vi "AlliGator Compute Lifetime Variances.vi"(8 "error in (no error)":errorcluster, 10 "Lifetime Variance Data Array (in)":T2[](array[typedef]), 11 "Slices Definition":T3={"Axis Start"=0.0, "Axis Stop"=0.0, "# Steps"=0, "Step Size"=0.0, "Step Definition"=enum."# Steps", "Upper Percentile"=0.0, "Lower Percentile"=0.0, "Min # Data Points/Slice"=0, "Output Abscissa Statistics Plots"=FALSE, "Bin Location"=enum."Left", "# Elements"=1, "Bootstrap CV's SDV"=FALSE, "# Replicas"=1} {"# Replicas" min=1; "# Elements" min=0; "Min # Data Points/Slice" min=1; "Lower Percentile" min=0.0 max=100.0; "Upper Percentile" min=0.0 max=100.0; "Step Size" min=0.0; "# Steps" min=1}) -> (0 "error out":errorcluster, 1 "Parameter Map Names":string[](array[string]), 2 "Lifetime Variance Data Array (out)":T2[](array[typedef]))   [LabVIEW 2021, in "AlliGator Decay Fit Parameter Map.lvlib"]
uses:
  AlliGator Decay Fit Parameter Map.lvlib
  Camera Noise Influence on Lifetime/Lifetime Variance Data.ctl
  Graphs/XY Graph/XY Graph Sliced Mean & SDV Step Definition.ctl
  Lifetime & Other Parameters/AlliGator Intensity Slice Definition.ctl
  Graphs/XY Graph/XY Graph Sliced CV Abscissa Location.ctl
  AlliGator Lifetime Variance Statistical Test.ctl
  Lifetime & Other Parameters/AlliGator Lifetime & Other Parameters.lvlib
  Graphs/XY Graph/XY Graph Add-Ons.lvlib
panel:
  in  "Variance Statistical Test":T1
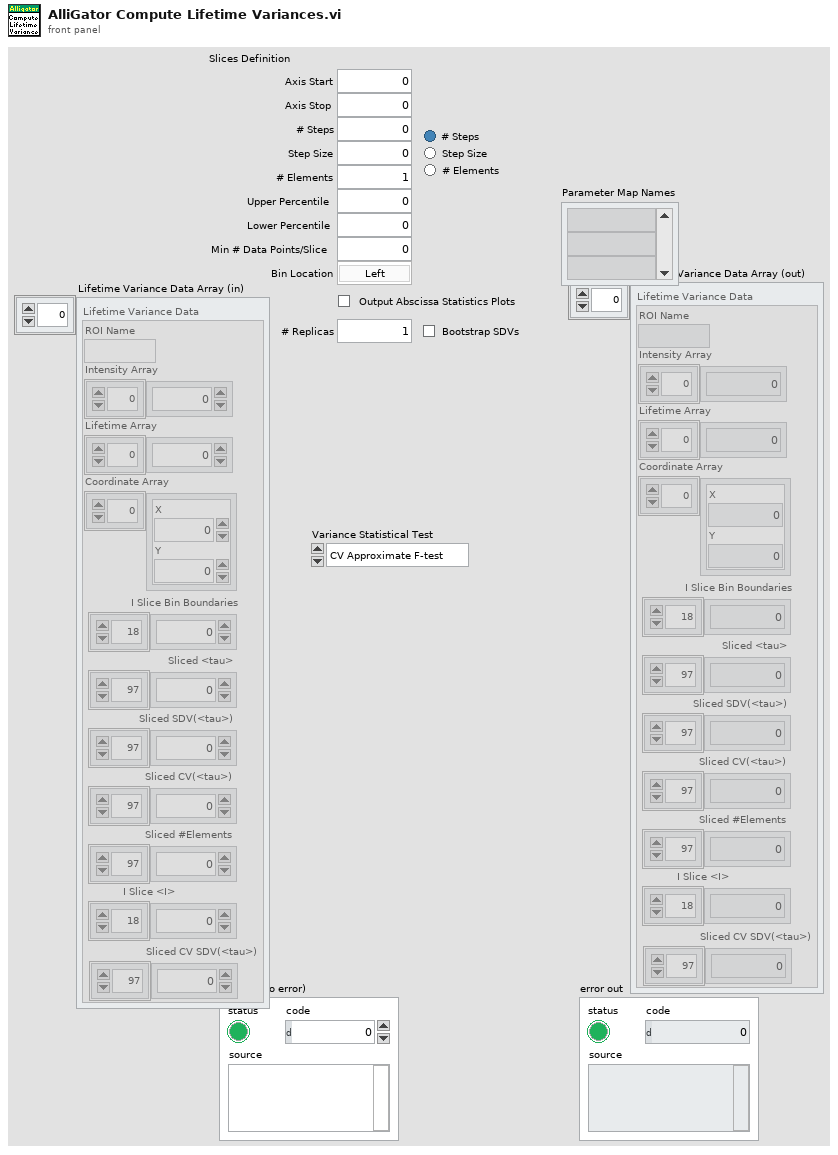
[diagram p1: front panel]
types:
  T1 = typedef "AlliGator Decay Fit Parameter Map.lvlib/AlliGator Lifetime Variance Statistical Test.ctl" = enum16{"CV Approximate F-test", "Variance F-test", "CV Residuals test", "CV Bootstrap SDV Test"}
  T2 = typedef "AlliGator Decay Fit Parameter Map.lvlib/Lifetime Variance Data.ctl" = cluster{"ROI Name":string, "Intensity Array":sgl[], "Lifetime Array":dbl[], "Coordinate Array":cluster{"X":i32, "Y":i32}[], "I Slice Bin Boundaries":dbl[], "Sliced <tau>":dbl[], "Sliced SDV(<tau>)":dbl[], "Sliced CV(<tau>)":dbl[], "Sliced #Elements":i32[], "I Slice <I>":dbl[], "Sliced CV SDV(<tau>)":dbl[]}
  T3 = typedef "XY Graph Add-Ons.lvlib/XY Graph Sliced Mean & SDV Step Definition.ctl" = cluster{"Axis Start":dbl, "Axis Stop":dbl, "# Steps":i32, "Step Size":dbl, "Step Definition":T4, "Upper Percentile":dbl, "Lower Percentile":dbl, "Min # Data Points/Slice":i32, "Output Abscissa Statistics Plots":bool, "Bin Location":T5, "# Elements":i32, "Bootstrap CV's SDV":bool, "# Replicas":i32}
  T4 = typedef "AlliGator Lifetime & Other Parameters.lvlib/AlliGator Intensity Slice Definition.ctl" = enum32{"# Steps", "Step Size", "# Elements"}
  T5 = typedef "XY Graph Add-Ons.lvlib/XY Graph Sliced CV Abscissa Location.ctl" = enum16{"Left", "Center", "Mean", "Right"}
  T6 = cluster{"Intensity Array":sgl[], "Lifetime Array":dbl[]}
  T7 = typedef "AlliGator Decay Fit Parameter Map.lvlib/AlliGator Sliced Analysis Plots.ctl" = cluster{"[<tau>(I)]":T8, "[SDV(tau)(I)]":T8, "[CV(tau)(I)]":T8, "[CV(tau)(I) SDV]":T8, "[N(I)]":T8, "[<I>(I)]":T8, "[SDV(I)(I)]":T8}
  T8 = typedef "XY Graph Add-Ons.lvlib/XY Graph Plot Data.ctl" = cluster{"X Array":dbl[], "Y Array":dbl[]}
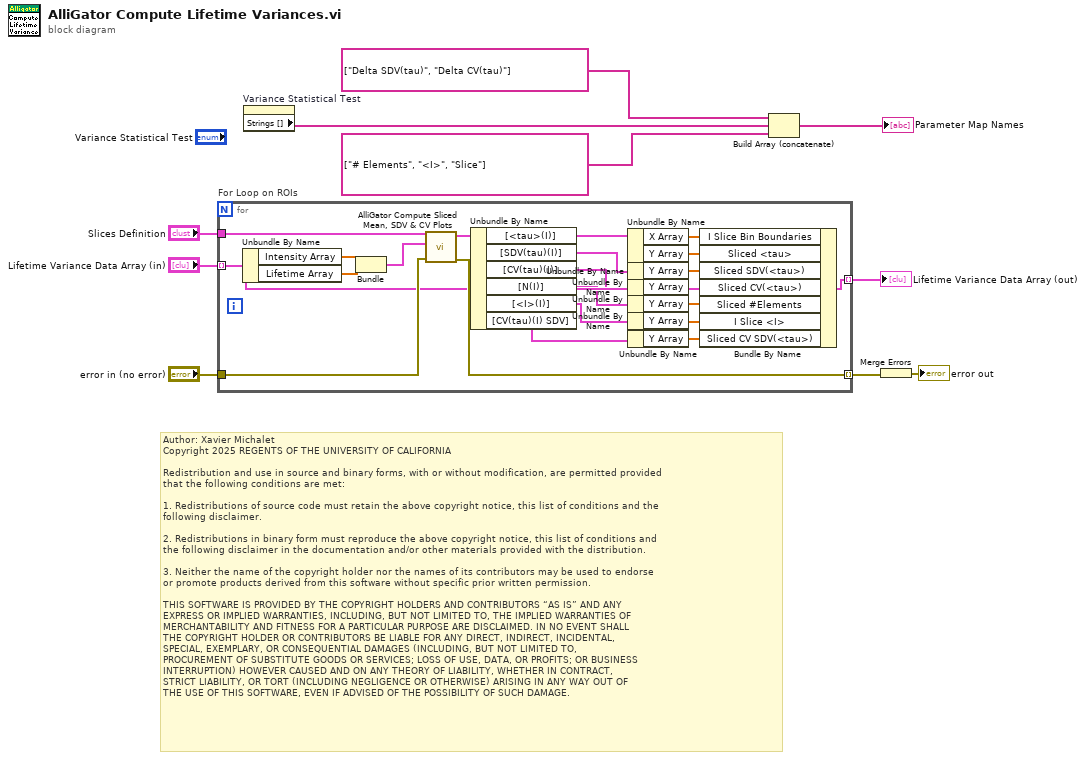
[diagram p0: block diagram]
diagram:
  # "Author: Xavier Michalet\nCopyright 2025 REGENTS OF THE UNIVERSITY OF CALIFORNIA\n\nRedistribution and use in source and binary forms, with or without modification, are permitted provided\nthat the following conditions are met:\n\n1. Redistributions of source code must retain the above copyright notice, this list of conditions and the\nfollowing disclaimer.\n\n2. Redistributions in binary form must reproduce the above copyright notice, this list of conditions and\nthe following disclaimer in the documentation and/or other materials provided with the distribution.\n\n3. Neither the name of the copyright holder nor the names of its contributors may be used to endorse \nor promote products derived from this software without specific prior written permission.\n\nTHIS SOFTWARE IS PROVIDED BY THE COPYRIGHT HOLDERS AND CONTRIBUTORS “AS IS” AND ANY \nEXPRESS OR IMPLIED WARRANTIES, INCLUDING, BUT NOT LIMITED TO, THE IMPLIED WARRANTIES OF\nMERCHANTABILITY AND FITNESS FOR A PARTICULAR PURPOSE ARE DISCLAIMED. IN NO EVENT SHALL\nTHE COPYRIGHT HOLDER OR CONTRIBUTORS BE LIABLE FOR ANY DIRECT, INDIRECT, INCIDENTAL, \nSPECIAL, EXEMPLARY, OR CONSEQUENTIAL DAMAGES (INCLUDING, BUT NOT LIMITED TO, \nPROCUREMENT OF SUBSTITUTE GOODS OR SERVICES; LOSS OF USE, DATA, OR PROFITS; OR BUSINESS\nINTERRUPTION) HOWEVER CAUSED AND ON ANY THEORY OF LIABILITY, WHETHER IN CONTRACT, \nSTRICT LIABILITY, OR TORT (INCLUDING NEGLIGENCE OR OTHERWISE) ARISING IN ANY WAY OUT OF\nTHE USE OF THIS SOFTWARE, EVEN IF ADVISED OF THE POSSIBILITY OF SUCH DAMAGE."
  n1 = for "For Loop on ROIs" {
    tunnel: "Slices Definition" -> [w32]
    tunnel: "Lifetime Variance Data Array (in)" -> [w26] mode=indexing
    tunnel: "error in (no error)" -> [w28]
    tunnel: [w27] -> w7 mode=indexing
    tunnel: [w23] -> w5 mode=indexing
    n2 = Unbundle By Name(w26) -> ("Intensity Array"=w31:sgl[], "Lifetime Array"=w30:dbl[])
    n3 = Bundle("Intensity Array"=w31, "Lifetime Array"=w30) -> (w29:T6)  [unwired: 1 in]
    n4 = call "AlliGator Compute Sliced Mean, SDV & CV Plots.vi"("error in (no error)"=w28, "tau(I) Plot"=w29, "Slices Definition"=w32) -> ("error out"=w27:errorcluster, "Result Plots Cluster"=w22:T7)  [unwired: 5 in, 2 out]
    n5 = Unbundle By Name(w22) -> ("[<tau>(I)]"=w21:T8, "[SDV(tau)(I)]"=w20:T8, "[CV(tau)(I)]"=w19:T8, "[N(I)]"=w18:T8, "[<I>(I)]"=w17:T8, "[CV(tau)(I) SDV]"=w12:T8)
    n6 = Unbundle By Name(w21) -> ("X Array"=w25:dbl[], "Y Array"=w24:dbl[])
    n7 = Unbundle By Name(w20) -> ("Y Array"=w16:dbl[])
    n8 = Unbundle By Name(w19) -> ("Y Array"=w15:dbl[])
    n9 = Unbundle By Name(w18) -> ("Y Array"=w14:dbl[])
    n10 = Unbundle By Name(w17) -> ("Y Array"=w13:dbl[])
    n11 = Unbundle By Name(w12) -> ("Y Array"=w11:dbl[])
    n12 = Bundle By Name(cluster=w26, "I Slice Bin Boundaries"=w25, "Sliced <tau>"=w24, "Sliced SDV(<tau>)"=w16, "Sliced CV(<tau>)"=w15, "Sliced #Elements"=w14, "I Slice <I>"=w13, "Sliced CV SDV(<tau>)"=w11) -> (w23:T2)
  }
  "Lifetime Variance Data Array (out)" <- w5
  n13 = property on="Variance Statistical Test" class="Enum (strict)"() -> ("Strings []"=w2:string[])  [unwired: 2 in, 2 out]
  n14 = Build Array (concatenate)(string[] ["Delta SDV(tau)", "Delta CV(tau)"] ("Parameter Map Names"), w2, string[] ["# Elements", "<I>", "Slice"] ("Parameter Map Names")) -> (→"Parameter Map Names":string[])
  n15 = Merge Errors(w7) -> (→"error out":errorcluster)
